vi "FPGAMain.vi"() -> ()   [LabVIEW 2013]
uses:
  <vilib>/Platform/TimedLoop/XDataNode/timing_clust.ctl
  <vilib>/Platform/TimedLoop/XDataNode/nitl_modes.ctl
  <vilib>/Platform/TimedLoop/XDataNode/wakeup.ctl
  <vilib>/rvi/Emulation/niFpgaSctlEmulationGetInTimedLoop.vi
  <vilib>/rvi/Emulation/niFpgaEmulationReportErrorSimple.vi
  <vilib>/rvi/Emulation/niFpgaGetClockAttributes.vi
  <vilib>/rvi/eio/common/nirviEmuTemplateMethod_errors.vi
  <vilib>/rvi/Emulation/niFpgaCriticalErrorInLSC.vi
  <vilib>/rvi/Emulation/niFpgaProcessEmulError.vi
  <vilib>/Platform/TimedLoop/XDataNode/XDataNode.xnode
  <vilib>/eio/EIONode/EIONode.xnode
  <vilib>/Platform/TimedLoop/XDataNode/XDNodeRunTimeDep.lvlib
panel:
  out "Width(ticks)":u64
  in  "TrigPulseWidthMin(ticks)":u64
  in  "ArmTrigger":bool
  out "TriggerFired":bool
  in  "ResetTrigger":bool
  out "TriggerArmed":bool
  in  "TriggerAutoReArm(mSec)":i64=-1
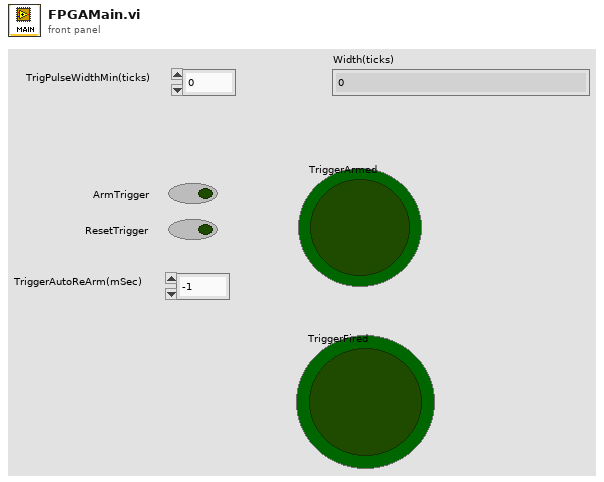
[diagram p1: front panel]
types:
  T1 = typedef "XDNodeRunTimeDep.lvlib/timing_clust.ctl" = cluster{"Expected End [f-1]":u64, "Actual End [f-1]":u64, "Finished Late? [f-1]":bool, "Expected End [i-1]":u64, "Actual End [i-1]":u64, "Finished Late? [i-1]":bool, "Expected Start [i]":u64, "Actual Start [i]":u64, "Expected Start [f]":u64, "Actual Start [f]":u64, "Source Name":string, "Structure Name":string, "Period":i64, "Deadline":i64, "Offset":i64, "Start":i64, "Priority":i32, "Timeout":i32, "Mode":T2, "Wakeup Reason":T3, "Error":errorcluster, "Source Type":string, "Secondary Source Type":string, "Global End Time":u64, "Global Start Time":u64, "Frame Duration":u64, "Iteration Duration":u64, "Assigned CPU":i32, "I/O Scan Engine Mode":u32}
  T2 = typedef "XDNodeRunTimeDep.lvlib/nitl_modes.ctl" = enum32{"No Change", "Process missed periods, maintain original phase", "Discard missed periods, maintain original phase", "Process missed periods, ignore original phase", "Discard missed periods, ignore original phase"}
  T3 = typedef "XDNodeRunTimeDep.lvlib/wakeup.ctl" = enum32{"Normal", "Aborted", "Asynchronous wakeup", "Timing source error", "Timed loop error", "Timeout"}
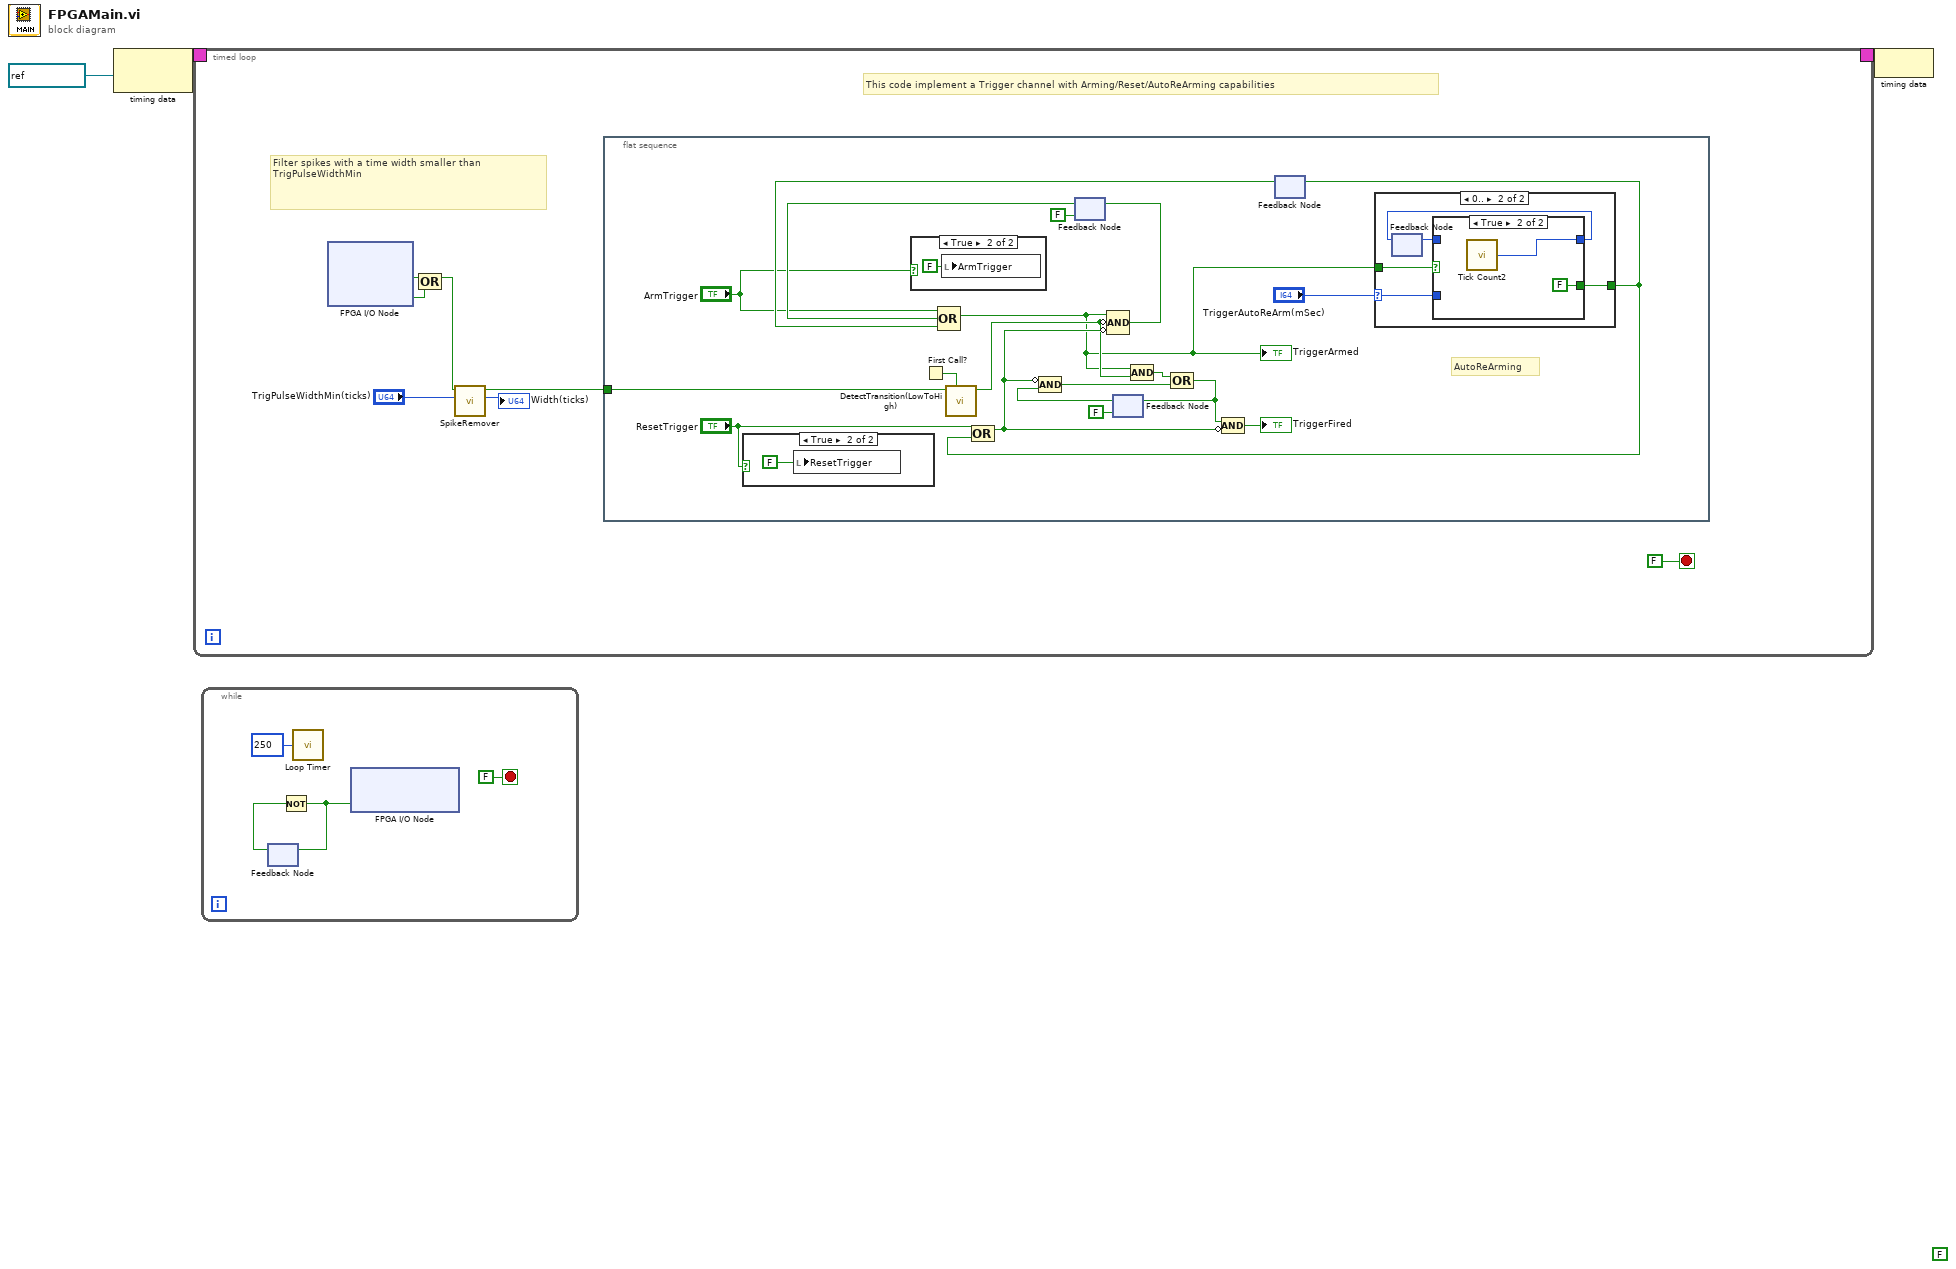
[diagram p0: block diagram]
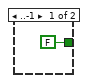
[diagram p4: hidden frame]
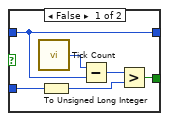
[diagram p5: hidden frame]
diagram:
  (unwired) FALSE
  n1 = node-c288(refnum<k21> "80MHz" ("Source Name")) -> (w2:T1)
  n2 = timed-loop {
    timing: w2 -> [_]
    timing-out: [_] -> w1
    stop <- FALSE stop-if-true
    # "This code implement a Trigger channel with Arming/Reset/AutoReArming capabilities"
    # "Filter spikes with a time width smaller than TrigPulseWidthMin"
    n3 = xnode "FPGA I/O Node"() -> ("DIO12"=w6:bool, "DIO0"=w4:bool)  [unwired: 2 in, 2 out]
    n4 = Compound Arithmetic op=OR(w6, w4) -> (w5:bool)
    n5 = call "SpikeRemover.vi"("TrigPulseWidthMin(ticks)"="TrigPulseWidthMin(ticks)", "TriggerIn"=w5) -> ("MEasuredPulseWidth"=→"Width(ticks)":u64, "FilteredTrigger"=w8:bool)  [unwired: 8 in]
    n6 = flat-sequence {
      tunnel: w8 -> [w11]
      frame #0 {
        # "AutoReArming"
        n7 = case shown="True" "ResetTrigger" {
          frame False {
          }
          frame True {
            n8 = local write "ResetTrigger"(FALSE ("ResetTrigger")) -> ()
          }
        }
        n9 = case shown="True" "ArmTrigger" {
          frame False {
          }
          frame True {
            n10 = local write "ArmTrigger"(FALSE ("ResetTrigger")) -> ()
          }
        }
        n11 = First Call?() -> (First Call?: T/F=w17:bool)
        n12 = call "DetectTransition(LowToHigh).vi"("First Call?: T/F"=w17, "InputSignal"=w11) -> ("RaisingFrontDetected"=w16:bool)  [unwired: 9 in]
        n13 = feedback #1(FALSE) -> (w29:bool)
        n14 = feedback #2(FALSE) -> (w23:bool)
        n15 = feedback #3() -> (w21:bool)  [unwired: 1 in]
        n16 = Compound Arithmetic op=OR("ArmTrigger", w29, w21) -> (w15:bool)
        "TriggerArmed" <- w15
        n17 = Compound Arithmetic op=AND(w15, w16) -> (w22:bool)
        n18 = case shown="0.." "TriggerAutoReArm(mSec)" {
          selector: "TriggerAutoReArm(mSec)" -> [_ w34]
          tunnel: [FALSE w33] -> w12
          tunnel: w15 -> [_ w35]
          frame ..-1 {
          }
          frame 0.. {
            n19 = feedback #4() -> (w36:u32)  [unwired: 1 in]
            n20 = case shown="True" w35 {
              tunnel: [w42 w45] -> w37
              tunnel: w36 -> [w42 _]
              tunnel: w34 -> [w40 _]
              tunnel: [w39 FALSE] -> w33
              frame False {
                n21 = call "Tick Count"() -> ("Tick Count(mSec)"=w43:u32)
                n22 = To Unsigned Long Integer(number=w40) -> (unsigned 32bit integer=w38:u32)
                n23 = Subtract(x=w43, y=w42) -> (x-y=w41:u32)
                n24 = Greater?(x=w41, y=w38) -> (0:w39:bool)
              }
              frame True {
                n25 = call "Tick Count2"() -> ("Tick Count(mSec)"=w45:u32)
              }
            }
            n26 = feedback-in #4(w37) -> ()
          }
        }
        n27 = Compound Arithmetic op=OR("ResetTrigger", w12) -> (w19:bool)
        n28 = Compound Arithmetic op=AND(invert w19, w23) -> (w24:bool)
        n29 = Compound Arithmetic op=AND(w15, invert w16, invert w19) -> (w28:bool)
        n30 = feedback-in #1(w28) -> ()
        n31 = Compound Arithmetic op=OR(w22, w24) -> (w26:bool)
        n32 = feedback-in #2(w26) -> ()
        n33 = Compound Arithmetic op=AND(w26, invert w19) -> (→"TriggerFired":bool)
        n34 = feedback-in #3(w12) -> ()
      }
    }
  }
  n35 = while {
    stop <- FALSE stop-if-true
    n36 = feedback #5() -> (w50:bool)  [unwired: 1 in]
    n37 = Not(x=w50) -> (.not. x?=w49:bool)
    n38 = feedback-in #5(w49) -> ()
    n39 = call "Loop Timer"("Count(mSec)"=u32 250) -> ()  [unwired: 1 out]
    n40 = xnode "FPGA I/O Node"("FPGA LED"=w49) -> ()  [unwired: 1 in, 1 out]
  }
  n41 = node-c288(w1) -> ()
